vi "Update Exp Auisitions.vi"(8 "error in (no error)":errorcluster, 11 "ExpVars":T1={"Experiment Type"="2D Snapshot", "Experiment Name"="Experiment_1", "ExpPath"=path "E:/Data", "TSFrames"=1000, "TSfps"=1000, "ZTSFrames"=1000, "ZTSdt"=1, "Streaming"=FALSE, "Z Stack Settings"={"Start"=0.0, "Step Size"=0.1, "Finish"=1.0}, "total images"=1, "tdms ref"=refnum, "frame #"=0, "images per stack"=1, "total stacks"=1, "period"=1, "PI MVR Increment"=""} {"period" min=1; "total stacks" min=1; "images per stack" min=1; "total images" min=1; "Z Stack Settings"."Start" min=0.0 max=100.0 step=0.1; "Z Stack Settings"."Step Size" min=0.1 max=100.0 step=0.1; "Z Stack Settings"."Finish" min=0.0 max=100.0 step=0.1; "TSFrames" min=1 step=1; "ZTSdt" min=1 step=1; "ZTSFrames" min=2 step=1; "TSfps" min=1 max=1000 step=1}) -> (0 "error out":errorcluster, 3 "ExpVars new #aqu":T1={"Experiment Type"="2D Snapshot", "Experiment Name"="Experiment_1", "ExpPath"=path "E:/Data", "TSFrames"=1000, "TSfps"=1000, "ZTSFrames"=1000, "ZTSdt"=1, "Streaming"=FALSE, "Z Stack Settings"={"Start"=0.0, "Step Size"=0.1, "Finish"=1.0}, "total images"=1, "tdms ref"=refnum, "frame #"=0, "images per stack"=1, "total stacks"=1, "period"=1, "PI MVR Increment"=""} {"period" min=1; "total stacks" min=1; "images per stack" min=1; "total images" min=1; "Z Stack Settings"."Start" min=0.0 max=100.0 step=0.1; "Z Stack Settings"."Step Size" min=0.1 max=100.0 step=0.1; "Z Stack Settings"."Finish" min=0.0 max=100.0 step=0.1; "TSFrames" min=1 step=1; "ZTSdt" min=1 step=1; "ZTSFrames" min=2 step=1; "TSfps" min=1 max=1000 step=1})   [LabVIEW 2020]
uses:
  _Controls/Exp Params.ctl
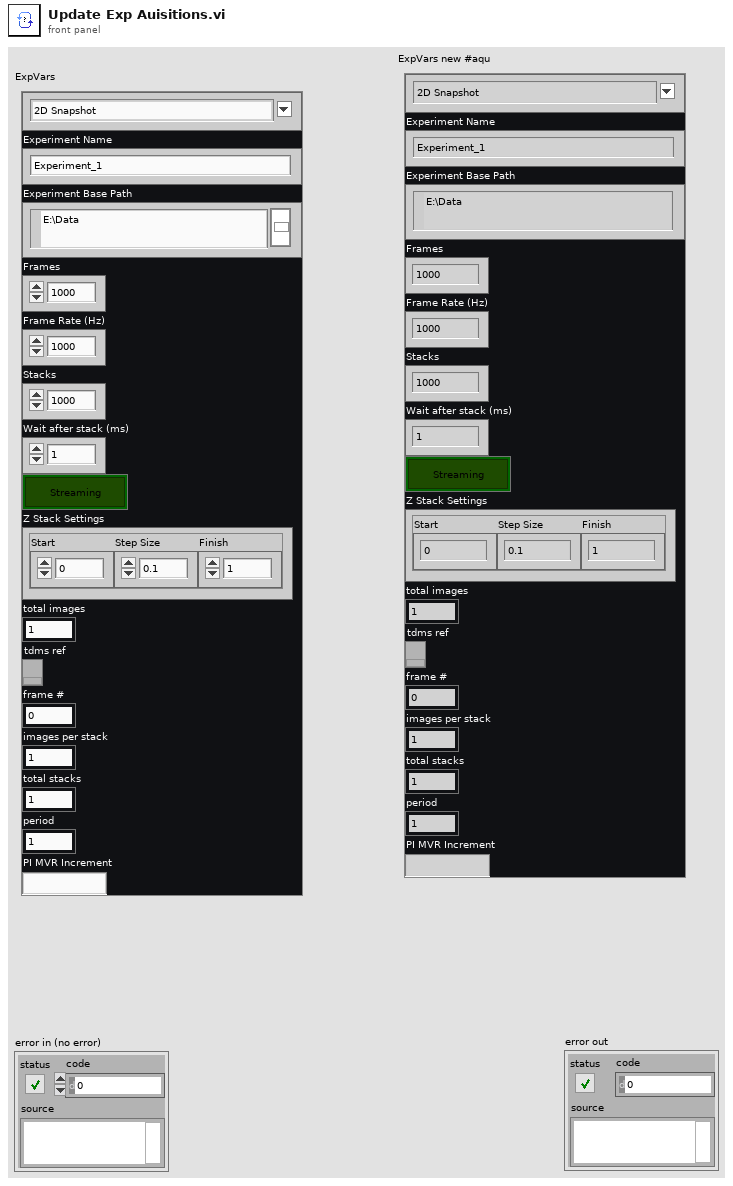
[diagram p1: front panel]
types:
  T1 = typedef "Exp Params.ctl" = cluster{"Experiment Type":string, "Experiment Name":string, "ExpPath":path, "TSFrames":i32, "TSfps":i32, "ZTSFrames":i32, "ZTSdt":i32, "Streaming":bool, "Z Stack Settings":cluster{"Start":dbl, "Step Size":dbl, "Finish":dbl}, "total images":i32, "tdms ref":refnum<k34>, "frame #":i64, "images per stack":i32, "total stacks":i32, "period":i32, "PI MVR Increment":string}
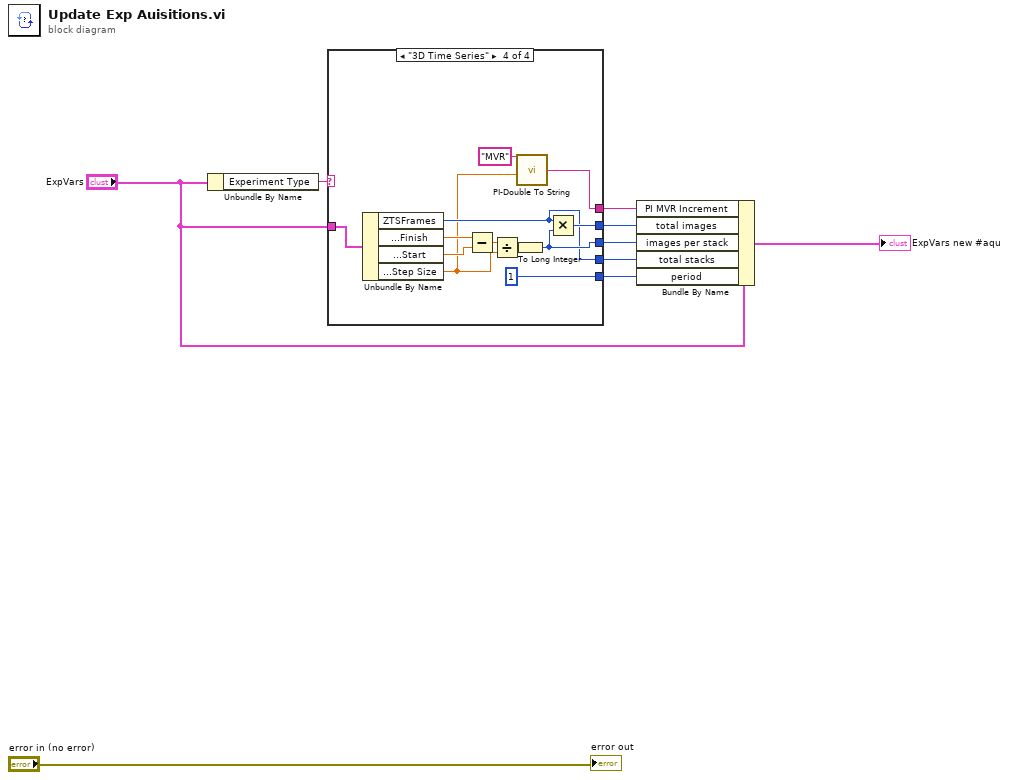
[diagram p0: block diagram]
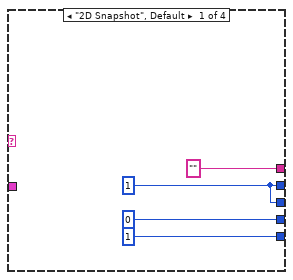
[diagram p2: hidden frame]
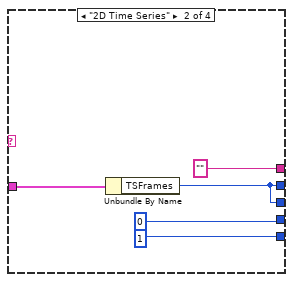
[diagram p3: hidden frame]
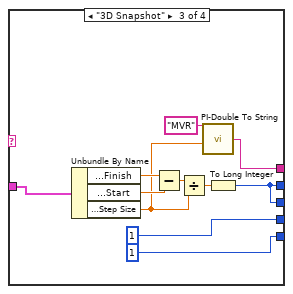
[diagram p4: hidden frame]
diagram:
  n1 = Unbundle By Name("ExpVars") -> ("Experiment Type"=w8:string)
  n2 = case shown="\"3D Time Series\"" w8 {
    tunnel: [w13 w17 w24 w36] -> w6
    tunnel: "ExpVars" -> [_ w18 w25 w37]
    tunnel: [0 ("# aquisitions") 0 ("# aquisitions") 1 ("# aquisitions") w34] -> w5
    tunnel: [w13 w17 w24 w35] -> w4
    tunnel: [1 ("# aquisitions") 1 ("# aquisitions") 1 ("# aquisitions") 1 ("# aquisitions")] -> w3
    tunnel: ["" "" w20 w31] -> w1
    frame "2D Snapshot", Default {
      w13 = 1 ("# aquisitions")
    }
    frame "2D Time Series" {
      n3 = Unbundle By Name(w18) -> ("TSFrames"=w17:i32)
    }
    frame "3D Snapshot" {
      n4 = Unbundle By Name(w25) -> ("Z Stack Settings.Finish"=w26:dbl, "Z Stack Settings.Start"=w28:dbl, "Z Stack Settings.Step Size"=w19:dbl)
      n5 = Subtract(x=w26, y=w28) -> (x-y=w27:dbl)
      n6 = Divide(x=w27, y=w19) -> (x/y=w29:dbl)
      n7 = call "PI-Double To String.vi"("Start"=w19, "String in"="MVR") -> ("String out"=w20:string)  [unwired: 2 in]
      n8 = To Long Integer(number=w29) -> (32bit integer=w24:i32)
    }
    frame "3D Time Series" {
      n9 = Unbundle By Name(w37) -> ("ZTSFrames"=w34:i32, "Z Stack Settings.Finish"=w38:dbl, "Z Stack Settings.Start"=w40:dbl, "Z Stack Settings.Step Size"=w30:dbl)
      n10 = Subtract(x=w38, y=w40) -> (x-y=w39:dbl)
      n11 = Divide(x=w39, y=w30) -> (x/y=w41:dbl)
      n12 = To Long Integer(number=w41) -> (32bit integer=w35:i32)
      n13 = call "PI-Double To String.vi"("Start"=w30, "String in"="MVR") -> ("String out"=w31:string)  [unwired: 2 in]
      n14 = Multiply(x=w34, y=w35) -> (x*y=w36:i32)
    }
  }
  n15 = Bundle By Name(cluster="ExpVars", "PI MVR Increment"=w1, "total images"=w6, "images per stack"=w4, "total stacks"=w5, "period"=w3) -> (→"ExpVars new #aqu":T1)
  "error out" <- "error in (no error)"
